vi "PRIME Detector Seperate Frames.vi"(8 "error in (no error)":errorcluster, 11 "Status":T1) -> (0 "error out":errorcluster, 1 "Final Frames":cluster{string[]}[](array[cluster]), 2 "Inter Frames":cluster{"CAMERA3":string[]}[](array[cluster]), 3 "Exp Frames":cluster{"CAMERA3":string[]}[](array[cluster]))   [LabVIEW 2024]
uses:
  PRIME Detector cluster Status.ctl
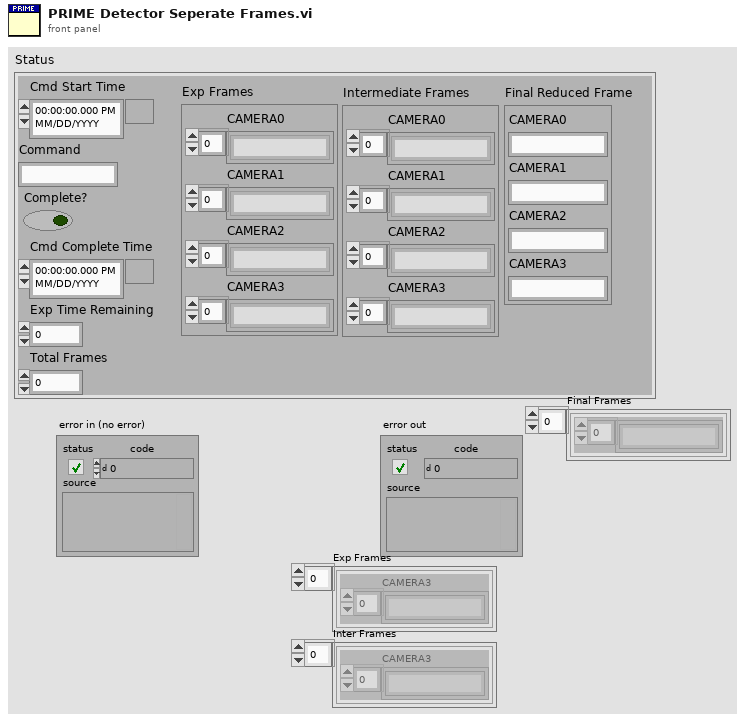
[diagram p1: front panel]
types:
  T1 = typedef "PRIME Detector cluster Status.ctl" = cluster{"Cmd Start Time":timestamp, "Command":string, "Complete?":bool, "Cmd Complete Time":timestamp, "Exp Time Remaining":dbl, "Total Frames":i32, "Exp Frames":cluster{"CAMERA0":string[], "CAMERA1":string[], "CAMERA2":string[], "CAMERA3":string[]}, "Intermediate Frames":cluster{"CAMERA0":string[], "CAMERA1":string[], "CAMERA2":string[], "CAMERA3":string[]}, "Final Reduced Frame":cluster{"CAMERA0":string, "CAMERA1":string, "CAMERA2":string, "CAMERA3":string}}
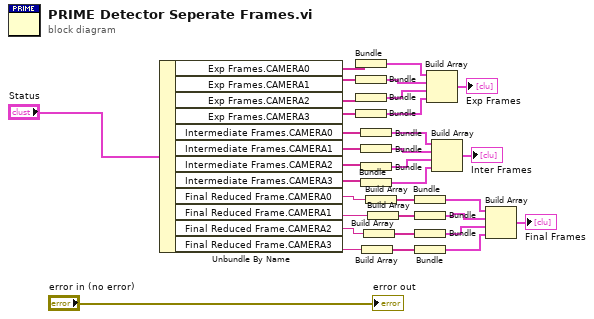
[diagram p0: block diagram]
diagram:
  n1 = Unbundle By Name("Status") -> ("Exp Frames.CAMERA0"=w28:string[], "Exp Frames.CAMERA1"=w27:string[], "Exp Frames.CAMERA2"=w26:string[], "Exp Frames.CAMERA3"=w25:string[], "Intermediate Frames.CAMERA0"=w19:string[], "Intermediate Frames.CAMERA1"=w18:string[], "Intermediate Frames.CAMERA2"=w17:string[], "Intermediate Frames.CAMERA3"=w16:string[], "Final Reduced Frame.CAMERA0"=w10:string, "Final Reduced Frame.CAMERA1"=w9:string, "Final Reduced Frame.CAMERA2"=w8:string, "Final Reduced Frame.CAMERA3"=w7:string)
  n2 = Bundle("CAMERA0"=w28) -> (w32:cluster{"CAMERA0":string[]})  [unwired: 1 in]
  n3 = Bundle("CAMERA1"=w27) -> (w31:cluster{"CAMERA1":string[]})  [unwired: 1 in]
  n4 = Bundle("CAMERA2"=w26) -> (w30:cluster{"CAMERA2":string[]})  [unwired: 1 in]
  n5 = Bundle("CAMERA3"=w25) -> (w29:cluster{"CAMERA3":string[]})  [unwired: 1 in]
  n6 = Bundle("CAMERA0"=w19) -> (w20:cluster{"CAMERA0":string[]})  [unwired: 1 in]
  n7 = Bundle("CAMERA1"=w18) -> (w21:cluster{"CAMERA1":string[]})  [unwired: 1 in]
  n8 = Bundle("CAMERA2"=w17) -> (w22:cluster{"CAMERA2":string[]})  [unwired: 1 in]
  n9 = Bundle("CAMERA3"=w16) -> (w23:cluster{"CAMERA3":string[]})  [unwired: 1 in]
  n10 = Build Array(w7) -> (w2:string[])
  n11 = Build Array(w8) -> (w3:string[])
  n12 = Build Array(w10) -> (w5:string[])
  n13 = Build Array(w9) -> (w4:string[])
  n14 = Bundle(w5) -> (w13:cluster{string[]})  [unwired: 1 in]
  n15 = Bundle(w4) -> (w6:cluster{string[]})  [unwired: 1 in]
  n16 = Bundle(w3) -> (w12:cluster{string[]})  [unwired: 1 in]
  n17 = Bundle(w2) -> (w11:cluster{string[]})  [unwired: 1 in]
  n18 = Build Array(w32, w31, w30, w29) -> (→"Exp Frames":cluster{"CAMERA3":string[]}[])
  n19 = Build Array(w20, w21, w22, w23) -> (→"Inter Frames":cluster{"CAMERA3":string[]}[])
  n20 = Build Array(w13, w6, w12, w11) -> (→"Final Frames":cluster{string[]}[])
  "error out" <- "error in (no error)"
